vi "FRCts20_Backend_Request_POST_reform.vi"(7 "Request":T1, 8 "error in (no error)":errorcluster, 11 "recordset data":variant[][](array[variant])) -> (0 "error out":errorcluster, 3 "data string":string)   [LabVIEW 2013]
uses:
  FRCts20_Backend_API/FRCts20_Backend_API_Request.ctl
  FRCts20_Backend_API/FRCts20_Backend_API_Status.ctl
  <vilib>/addons/database/_DB Variant To Data/Database Variant To Data.xnode
  FRCts20_Backend_Engine.lvlib
  FRCts20_Backend_API/FRCts20_Backend_API.lvlib
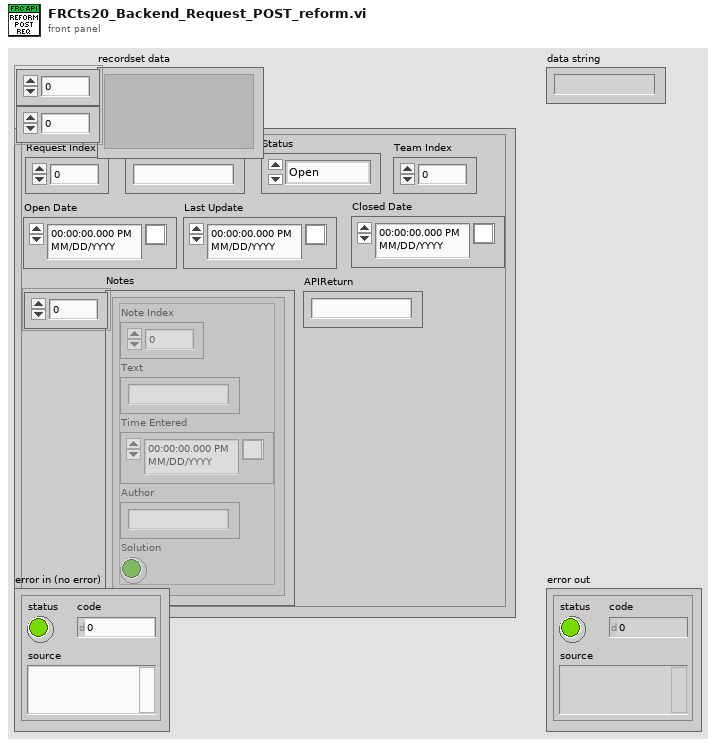
[diagram p1: front panel]
types:
  T1 = typedef "FRCts20_Backend_API.lvlib/FRCts20_Backend_API_Request.ctl" = cluster{"Request Index":u32, "Description":string, "Status":T2, "Open Date":timestamp, "Last Update":timestamp, "Closed Date":timestamp, "Notes":cluster{"Note Index":u32, "Text":string, "Time Entered":timestamp, "Author":string, "Solution":bool}[], "Team Index":u32, "APIReturn":string}
  T2 = typedef "FRCts20_Backend_API.lvlib/FRCts20_Backend_API_Status.ctl" = enum16{"Open", "In Work", "Closed"}
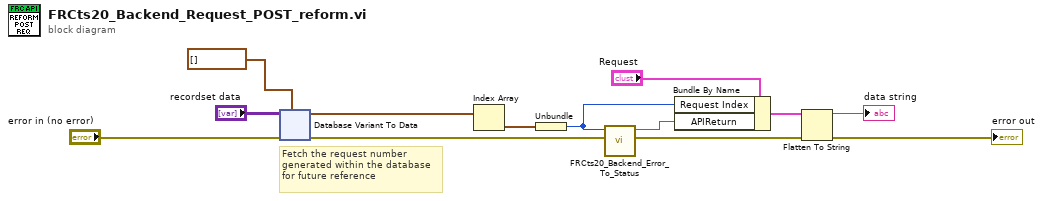
[diagram p0: block diagram]
diagram:
  # "Fetch the request number\ngenerated within the database\nfor future reference"
  n1 = xnode "Database Variant To Data"("database variant"="recordset data", "error in"="error in (no error)", "type"=cluster{u32}[] []) -> ("data"=w3:cluster{u32}[], "error out"=w9:errorcluster)
  n2 = Index Array(array=w3) -> (element=w4:cluster{u32})  [unwired: 1 in]
  n3 = Unbundle(w4) -> (w11:u32)
  n4 = call "FRCts20_Backend_Error_To_Status.vi"("error in (no error)"=w9, "rows affected"=w11) -> ("error out"=w10:errorcluster, "String"=w8:string)  [unwired: 8 in]
  n5 = Bundle By Name(cluster="Request", "Request Index"=w11, "APIReturn"=w8) -> (w5:T1)
  n6 = Flatten To String(anything=w5, error in (no error)=w10) -> (data string=→"data string":string, error out=→"error out":errorcluster)  [unwired: 2 in, 1 out]
